vi "Read Configuration File.vi"(8 "error in (no error)":errorcluster, 11 "FP-TC-Shared in":refnum<class "FP-TC-Shared.lvclass">) -> (0 "error out":errorcluster, 3 "FP-TC-Shared":refnum<class "FP-TC-Shared.lvclass">)   [LabVIEW 2019, in "FP-TC-Shared.lvclass"]
uses:
  FP-TC-Shared.lvclass
  C:/Program Files (x86)/National Instruments/LabVIEW 2019/user.lib/LevyLab/Instrument Framework/SMOs/Instrument/Instrument.lvclass
  <userlib>/LevyLab/Instrument Framework/SMOs/Instrument/Instrument.lvclass/Instrument.ctl
  <userlib>/LevyLab/Instrument Framework/SMOs/Configuration/Configuration.lvclass/Configuration.ctl
  FP-TC-Shared.lvclass/FP-TC-Shared.ctl
  <userlib>/LevyLab/Instrument Framework/SMOs/Configuration/Write Section.vi
  <userlib>/LevyLab/Instrument Framework/SMOs/Instrument/Instrument.lvclass
  C:/Program Files (x86)/National Instruments/LabVIEW 2019/vi.lib/JKI/JKI SMO/SMO/SMO.lvclass
  <vilib>/JKI/JKI SMO/SMO/Protected/ThisLevelClassName.vi
  <userlib>/LevyLab/Instrument Framework/SMOs/Configuration/Configuration.lvclass
  <userlib>/LevyLab/Instrument Framework/Instrument Types/Cryostat/Instrument.Cryostat.lvclass
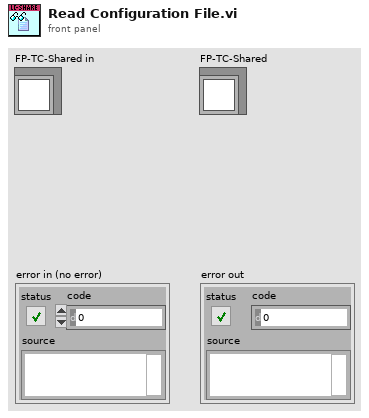
[diagram p1: front panel]
types:
  T1 = typedef "FP-TC-Shared.lvclass/LC Type--Enum.ctl" = enum16{"CF.TC", "CF.TC.Z", "CF.FP", "MNK.TC", "MNK.TC.Z", "MNK.FP"}
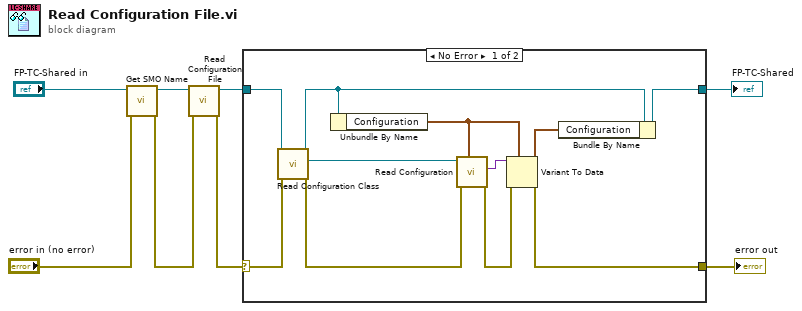
[diagram p0: block diagram]
diagram:
  n1 = call-dynamic "Get SMO Name.vi"("error in (no error)"="error in (no error)", "FP-TC-Shared in"="FP-TC-Shared in") -> ("error out"=w1:errorcluster, "FP-TC-Shared out"=w3:refnum<class "FP-TC-Shared.lvclass">)  [unwired: 7 in, 1 out]
  n2 = call-parent "Read Configuration File.vi"("error in (no error)"=w1, "Instrument in"=w3) -> ("error out"=w7:errorcluster, "Instrument out"=w8:refnum<class "FP-TC-Shared.lvclass">)  [unwired: 8 in]
  n3 = case shown="No Error" w7 {
    selector: w7 -> [w17 w21]
    tunnel: [w16 w21] -> w6
    tunnel: [w19 w20] -> w5
    tunnel: w8 -> [w18 w20]
    frame No Error {
      n4 = call <userlib>:"Read Configuration Class.vi"("error in (no error)"=w17, "Instrument in"=w18) -> ("error out"=w14:errorcluster, "Configuration"=w13:refnum<class "Configuration.lvclass">, "Instrument out"=w9:refnum<class "FP-TC-Shared.lvclass">)  [unwired: 7 in]
      n5 = Unbundle By Name(w9) -> ("Configuration"=w15:cluster{"LC Type":T1})
      n6 = call <userlib>:"Read Configuration.vi"("INI Fomatted Cluster Type"=w15, "error in (no error)"=w14, "Configuration in"=w13) -> ("error out"=w11:errorcluster, "Configuration"=w12:variant)  [unwired: 6 in, 1 out]
      n7 = Variant To Data(error in=w11, type=w15, Variant=w12) -> (data=w10:cluster{"LC Type":T1}, error out=w16:errorcluster)
      n8 = Bundle By Name(cluster=w9, "Configuration"=w10) -> (w19:refnum<class "FP-TC-Shared.lvclass">)
    }
    frame Error {
    }
  }
  "FP-TC-Shared" <- w5
  "error out" <- w6
